vi "Determine Trigger.vi"(5 "Detect?":bool[](array[boolean]), 7 "Command Indeces":T1, 8 "Time Since Last Generation":u32, 9 "Trigger":bool, 10 "Message Parameters":T3={"Generation Type"=enum."Trigger Only", "Period"=1.0, "Include Protection"=FALSE, "Type"=""}, 11 "Enabled":i32) -> (0 "Time Since Last Generation":u32, 1 "Trigger":bool)   [LabVIEW 2020, in "Instrument Addon Engine.lvlib"]
uses:
  Instrument Addon Engine.lvlib
  Addon Shared/Types/Message Parameters.ctl
  Addon Shared/Types/Message Generation Type.ctl
  Addon Shared/Types/Command Channel Indeces.ctl
  Addon Shared/Types/Command Channel Index.ctl
  Addon Shared/Instrument Addon Shared.lvlib
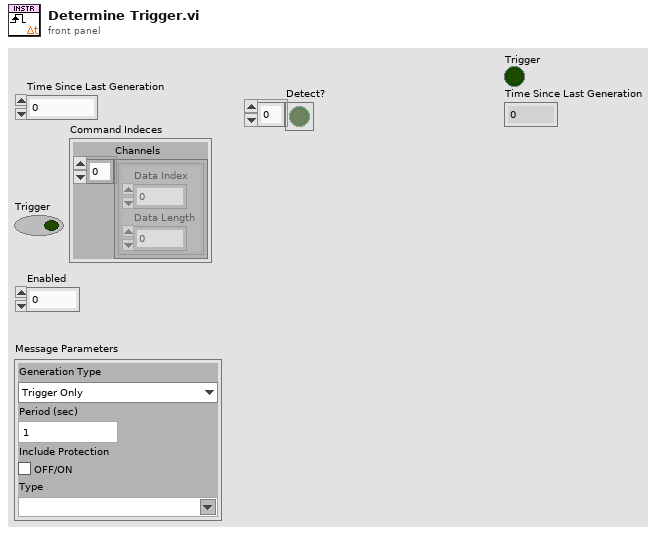
[diagram p1: front panel]
types:
  T1 = typedef "Instrument Addon Shared.lvlib/Command Channel Indeces.ctl" = cluster{"Channels":T2[]}
  T2 = typedef "Instrument Addon Shared.lvlib/Command Channel Index.ctl" = cluster{"Data Index":i32, "Data Length":i32}
  T3 = typedef "Instrument Addon Shared.lvlib/Message Parameters.ctl" = cluster{"Generation Type":T4, "Period":dbl, "Include Protection":bool, "Type":string}
  T4 = typedef "Instrument Addon Shared.lvlib/Message Generation Type.ctl" = enum16{"Trigger Only", "Periodic & Trigger", "Value Change & Trigger"}
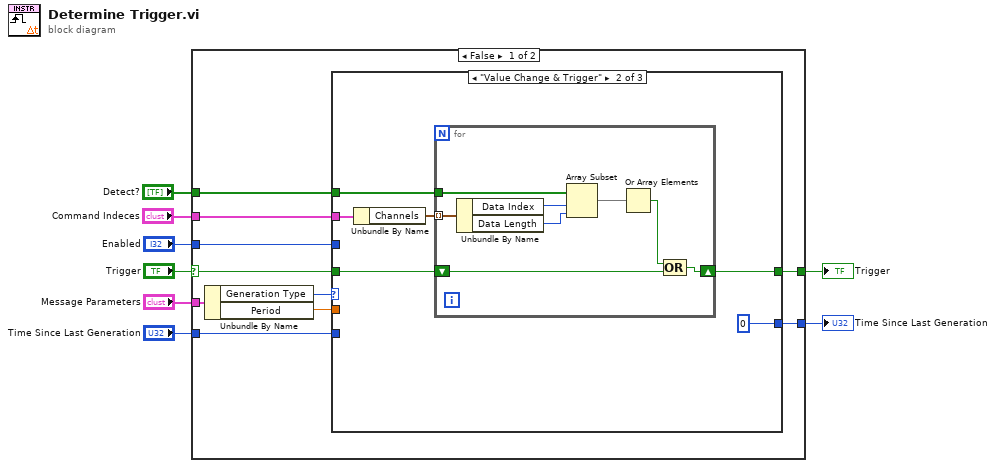
[diagram p0: block diagram]
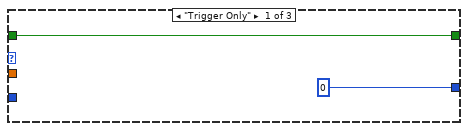
[diagram p2: hidden frame]
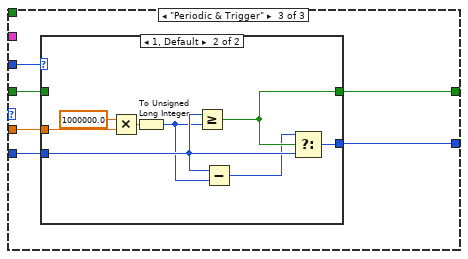
[diagram p3: hidden frame]
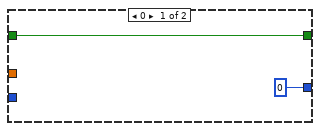
[diagram p4: hidden frame]
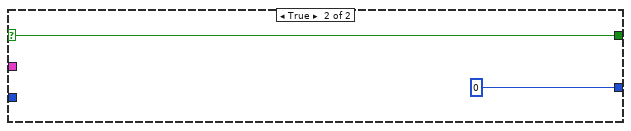
[diagram p5: hidden frame]
diagram:
  n1 = case shown="False" "Trigger" {
    selector: "Trigger" -> [w15 w52]
    tunnel: [w16 w52] -> w4
    tunnel: "Message Parameters" -> [w18 _]
    tunnel: "Enabled" -> [w14 _]
    tunnel: "Time Since Last Generation" -> [w12 _]
    tunnel: [w11 u32 0] -> w3
    tunnel: "Command Indeces" -> [w10 _]
    tunnel: "Detect?" -> [w9 _]
    frame False {
      n2 = Unbundle By Name(w18) -> ("Generation Type"=w17:T4, "Period"=w13:dbl)
      n3 = case shown="\"Value Change & Trigger\"" w17 {
        tunnel: [w20 w21 w39] -> w16
        tunnel: w15 -> [w20 w22 w38]
        tunnel: w14 -> [_ _ w40]
        tunnel: w13 -> [_ _ w37]
        tunnel: w12 -> [_ _ w36]
        tunnel: [u32 0 u32 0 w35] -> w11
        tunnel: w10 -> [_ w25 _]
        tunnel: w9 -> [_ w23 _]
        frame "Trigger Only" {
        }
        frame "Value Change & Trigger" {
          n4 = Unbundle By Name(w25) -> ("Channels"=w24:T2[])
          n5 = for {
            tunnel: w24 -> [w33] mode=indexing
            tunnel: w23 -> [w34]
            shift-right: [w27] -> w21
            shift-left: w22 -> [w28]
            n6 = Unbundle By Name(w33) -> ("Data Index"=w32:i32, "Data Length"=w31:i32)
            n7 = Array Subset(array=w34, index=w32, length=w31) -> (w30:bool[])
            n8 = Or Array Elements(Boolean array=w30) -> (logical OR=w29:bool)
            n9 = Compound Arithmetic op=OR(w29, w28) -> (w27:bool)
          }
        }
        frame "Periodic & Trigger" {
          n10 = case shown="1, Default" w40 {
            tunnel: [w42 w50] -> w39
            tunnel: w38 -> [w42 _]
            tunnel: w37 -> [_ w47]
            tunnel: w36 -> [_ w48]
            tunnel: [u32 0 w49] -> w35
            frame 0 {
            }
            frame 1, Default {
              n11 = Multiply(x=1000000.0, y=w47) -> (x*y=w45:dbl)
              n12 = To Unsigned Long Integer(number=w45) -> (unsigned 32bit integer=w43:u32)
              n13 = Greater Or Equal?(x=w48, y=w43) -> (x >= y?=w50:bool)
              n14 = Subtract(x=w48, y=w43) -> (x-y=w46:u32)
              n15 = Select(t=w46, s=w50, f=w48) -> (s? t:f=w49:u32)
            }
          }
        }
      }
    }
    frame True {
    }
  }
  "Trigger" <- w4
  "Time Since Last Generation" <- w3
